vi "Parse Sampler Data.vi"(8 "error in":errorcluster, 11 "Data":string) -> (0 "error out":errorcluster, 2 "Voltages (V)":dbl[](array[numeric]) format="%#_9g", 4 "Std. Dev. (V)":dbl, 6 "Mean (V)":dbl)   [LabVIEW 2019, in "ACSVcontrol-driver.lvlib"]
doc: "Parse data recieved from PJVS with sampler data."
uses:
  ACSVcontrol-driver.lvlib
  <vilib>/regexp/Match Regular Expression.xnode
  <vilib>/Analysis/NI_AALBase.lvlib
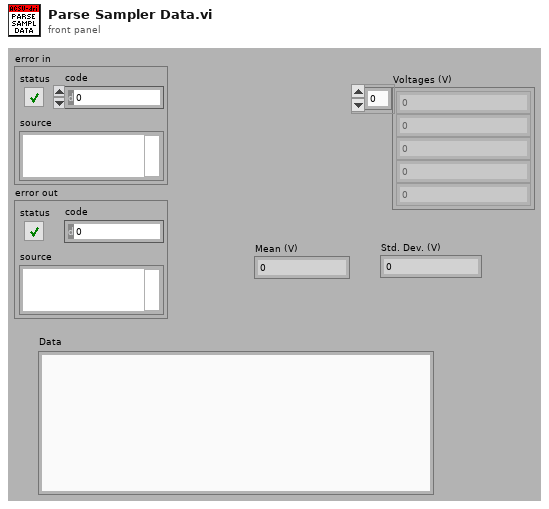
[diagram p1: front panel]
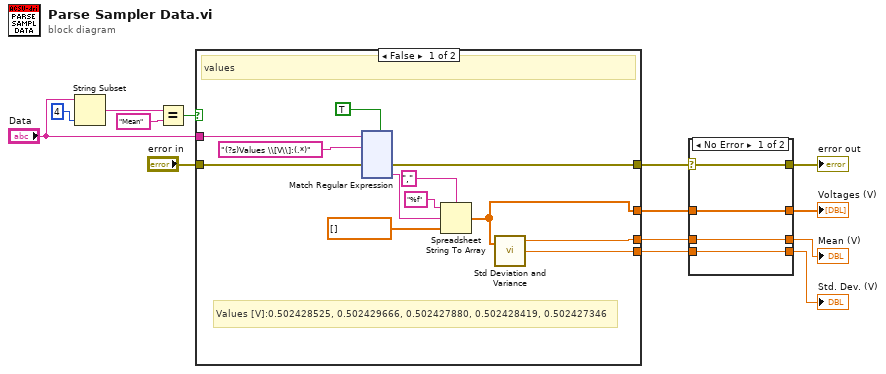
[diagram p0: block diagram]
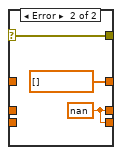
[diagram p2: hidden frame]
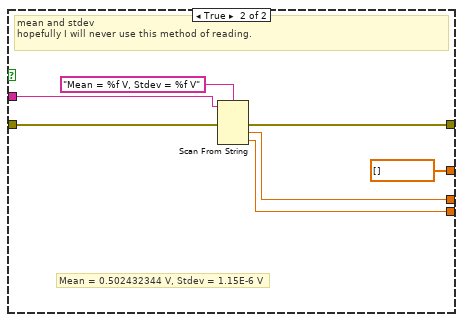
[diagram p3: hidden frame]
diagram:
  n1 = String Subset(string="Data", length (rest)=4 ("length (rest)")) -> (substring=w13:string)  [unwired: 1 in]
  n2 = Equal?(x=w13, y="Mean") -> (x = y?=w11:bool)
  n3 = case shown="False" w11 {
    tunnel: "Data" -> [w23 w148]
    tunnel: "error in" -> [w20 w147]
    tunnel: [w15 w146] -> w8
    tunnel: [w26 w145] -> w5
    tunnel: [w25 w144] -> w3
    tunnel: [w24 dbl[] [] ("array type (2D Dbl)")] -> w1
    frame False {
      # "Values [V]:0.502428525, 0.502429666, 0.502427880, 0.502428419, 0.502427346"
      # "values"
      n4 = xnode "Match Regular Expression"("input string"=w23, "regular expression"="(?s)Values \\[V\\]:(.*)", "error in"=w20, "multiline? (F)"=TRUE) -> ("error out"=w15:errorcluster, "submatch 1"=w16:string)  [unwired: 2 in, 4 out]
      n5 = Spreadsheet String To Array(delimiter (Tab)=",", format string="%f", spreadsheet string=w16, array type (2D Dbl)=dbl[] []) -> (array=w24:dbl[])
      n6 = call <vilib>:"Std Deviation and Variance.vi"("X"=w24) -> ("mean"=w26:dbl, "standard deviation"=w25:dbl)  [unwired: 1 in, 1 out]
    }
    frame True {
      # "Mean = 0.502432344 V, Stdev = 1.15E-6 V"
      # "mean and stdev\nhopefully I will never use this method of reading."
      n7 = Scan From String(format string="Mean = %f V, Stdev = %f V", input string=w148, error in=w147) -> (error out=w146:errorcluster, output 1=w145:dbl, output 2=w144:dbl)  [unwired: 3 in, 2 out]
    }
  }
  n8 = case shown="No Error" w8 {
    selector: w8 -> [w153 w156]
    tunnel: [w153 w156] -> w7
    tunnel: [w152 w154] -> w6
    tunnel: w5 -> [w152 _]
    tunnel: [w151 w154] -> w4
    tunnel: w3 -> [w151 _]
    tunnel: [w150 dbl[] [] ("array type (2D Dbl)")] -> w2
    tunnel: w1 -> [w150 _]
    frame No Error {
    }
    frame Error {
      w154 = nan
    }
  }
  "error out" <- w7
  "Mean (V)" <- w6
  "Std. Dev. (V)" <- w4
  "Voltages (V)" <- w2
